vi "Main.vi"() -> ()   [LabVIEW 2013, in "LinksApplication.lvclass"]
uses:
  LinksApplication.lvclass
  System.Windows.Forms
  Featherweight/Core/Actor/Instance/FTW-Actor.lvclass
  Featherweight/Core/Actor/Reference/FTW-ActorReference.lvclass
  Featherweight/Web/Utils/FTW-Web-HTTPResponseCode.ctl
  Featherweight/Core/Actor/Instance/FTW-Actor.lvclass/FTW-Actor.ctl
  Featherweight/Core/Sequencer/FTW-Sequencer.lvclass/FTW-Sequencer.ctl
  Featherweight/Core/Sequencer/FTW-SEQ-AddNext.vi
  Featherweight/Web/Server/FTW-WebService.lvclass
  <vilib>/wsapi/Web Request.lvclass
panel:
  in  "Top Level LabVIEW File":path caption="Select a LabVIEW File (VI, LVClass, LVLib) to analyze its static linkages"
  in  "Canvas":refnum<k24>(container)
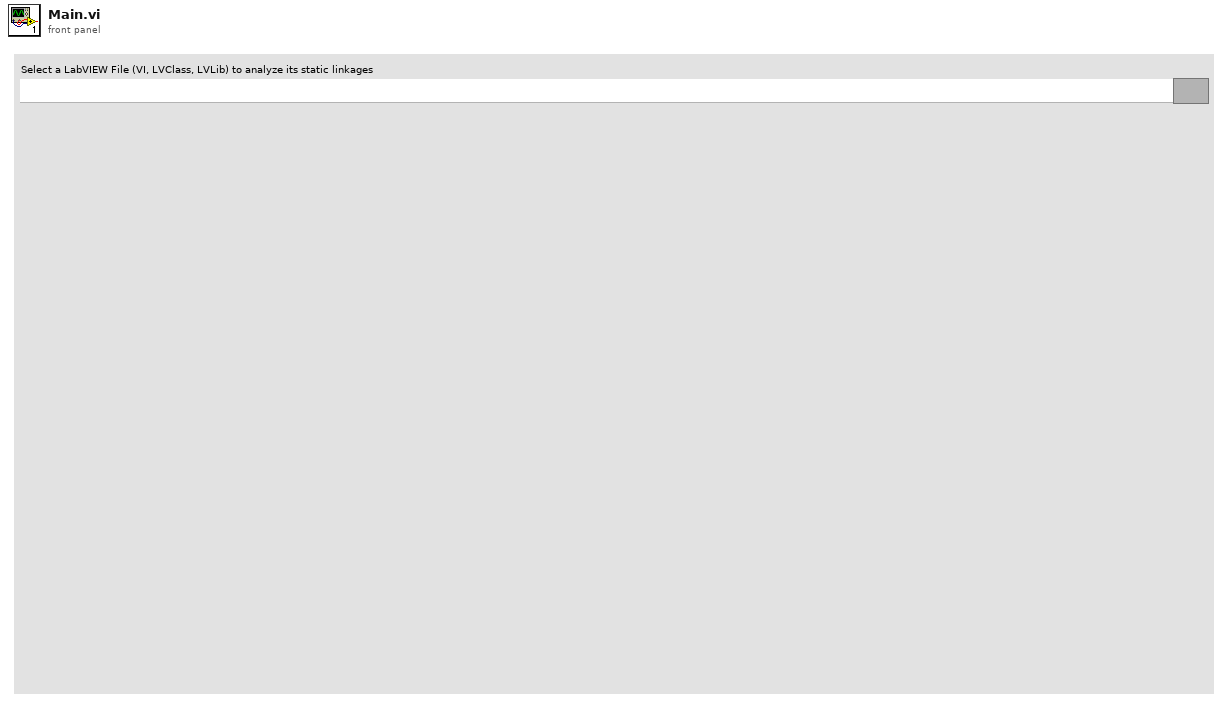
[diagram p1: front panel]
types:
  T1 = typedef "FTW-Web-HTTPResponseCode.ctl" = i32
  T2 = cluster{"Incoming HTTP Request":refnum<event-registration>}
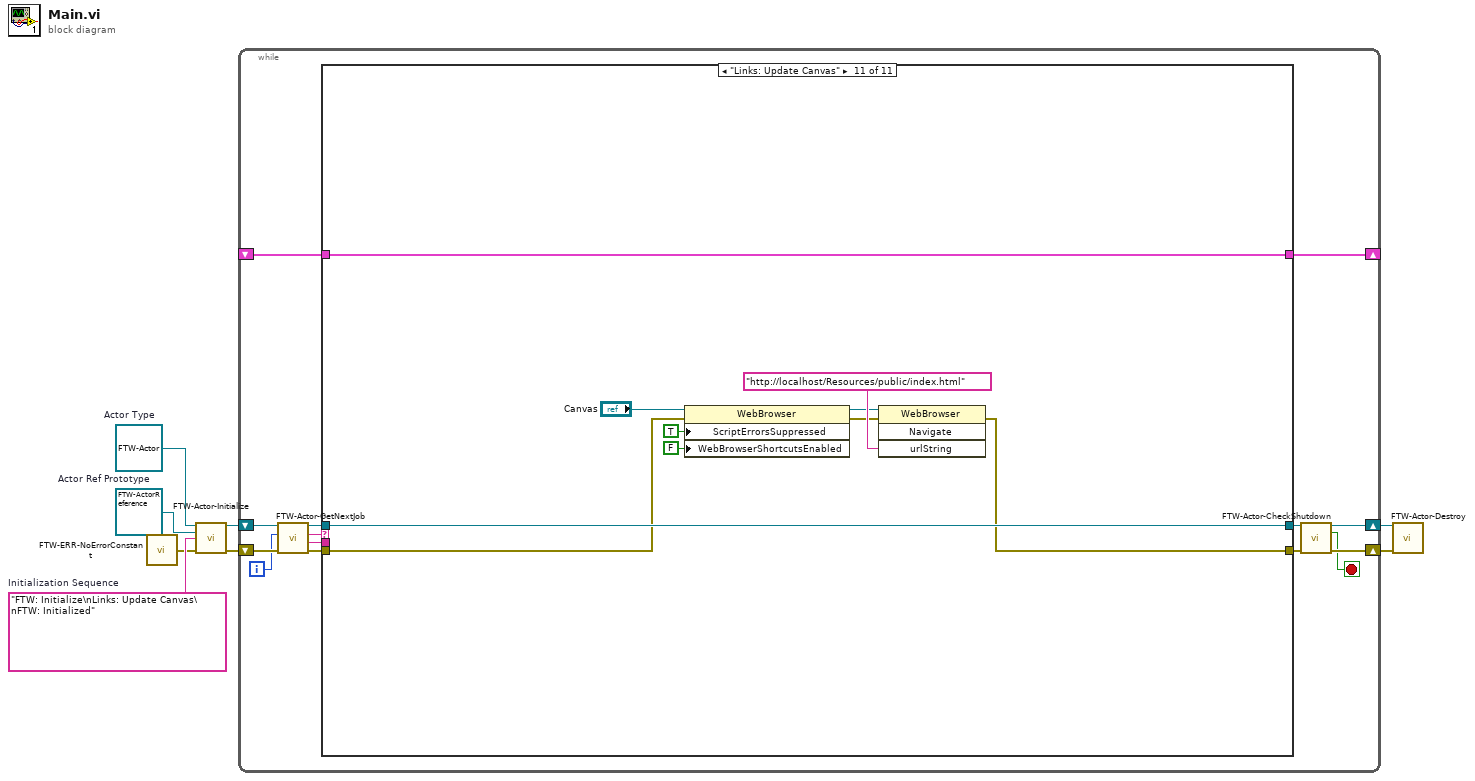
[diagram p0: block diagram]
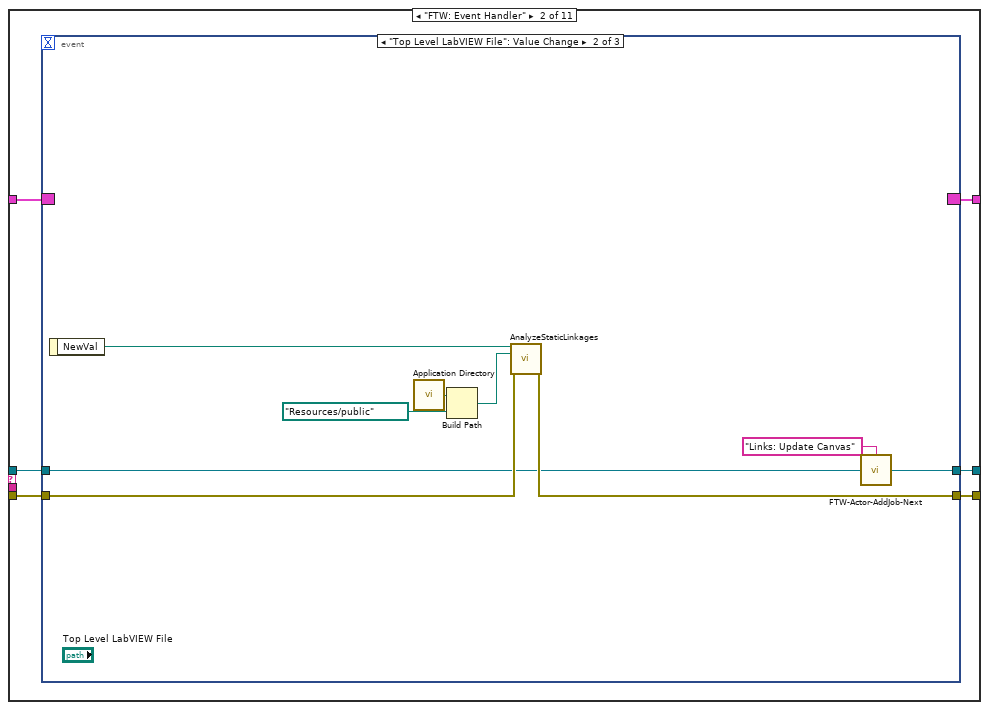
[diagram p3: hidden frame]
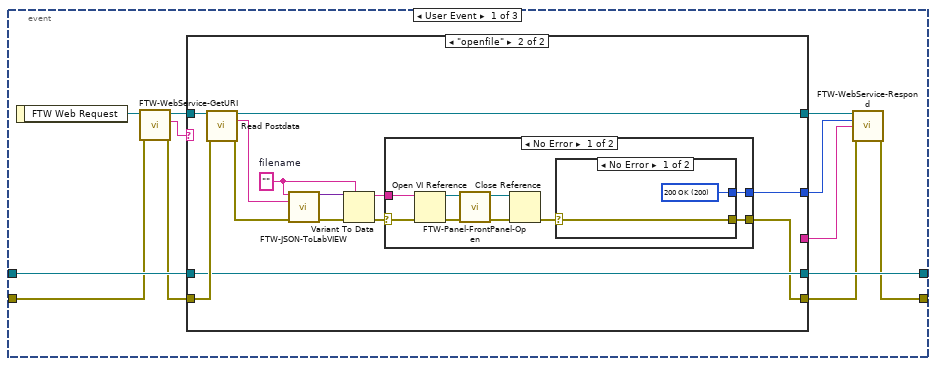
[diagram p4: hidden frame]
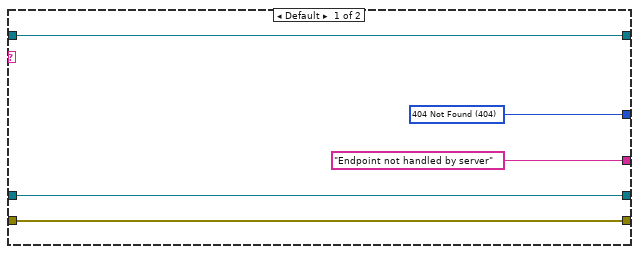
[diagram p5: hidden frame]
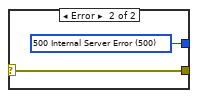
[diagram p6: hidden frame]
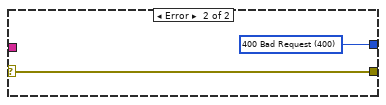
[diagram p7: hidden frame]
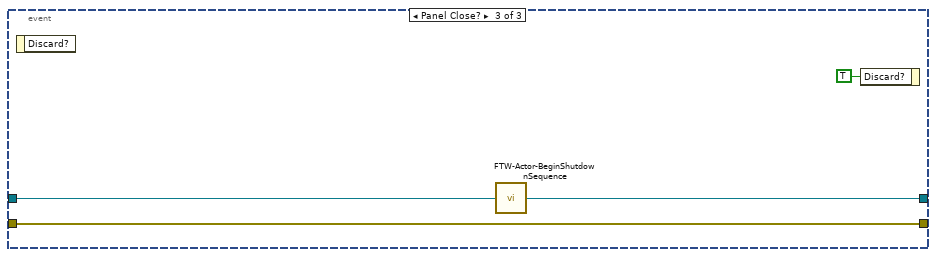
[diagram p8: hidden frame]
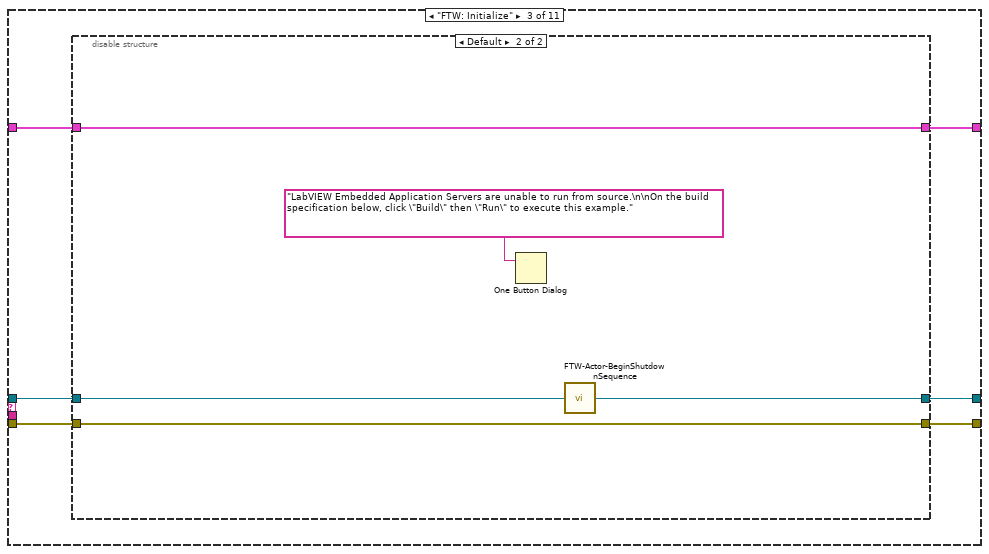
[diagram p9: hidden frame]
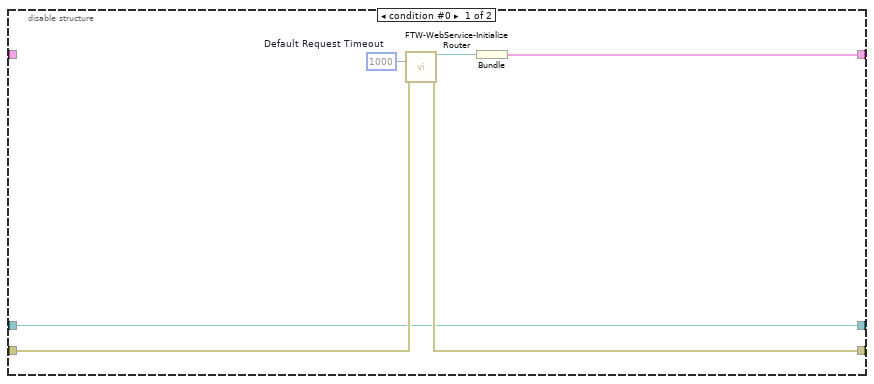
[diagram p10: hidden frame]
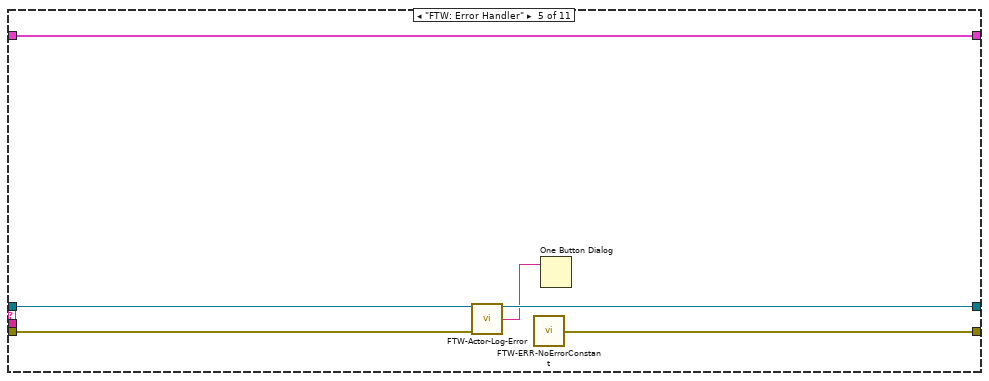
[diagram p12: hidden frame]
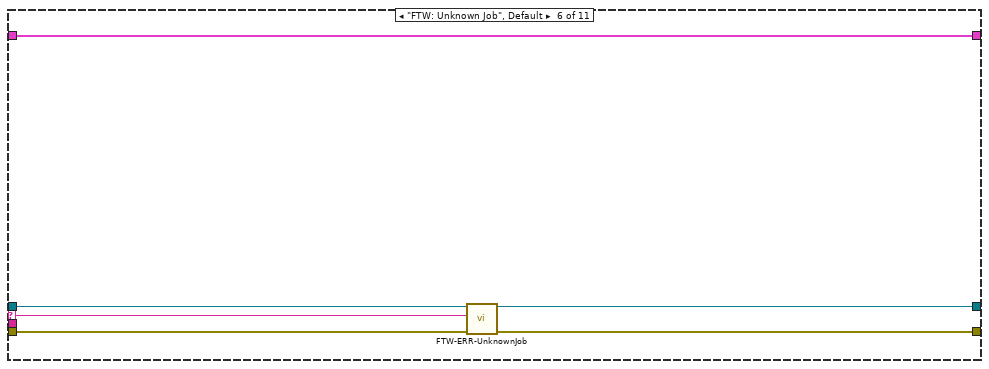
[diagram p13: hidden frame]
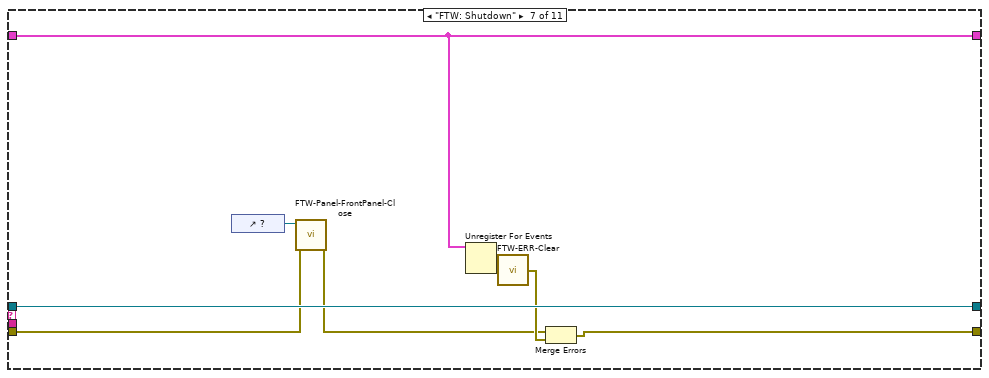
[diagram p14: hidden frame]
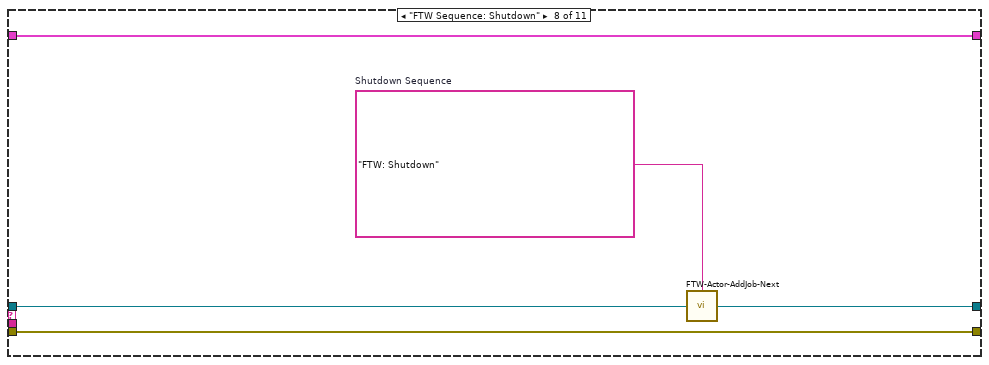
[diagram p15: hidden frame]
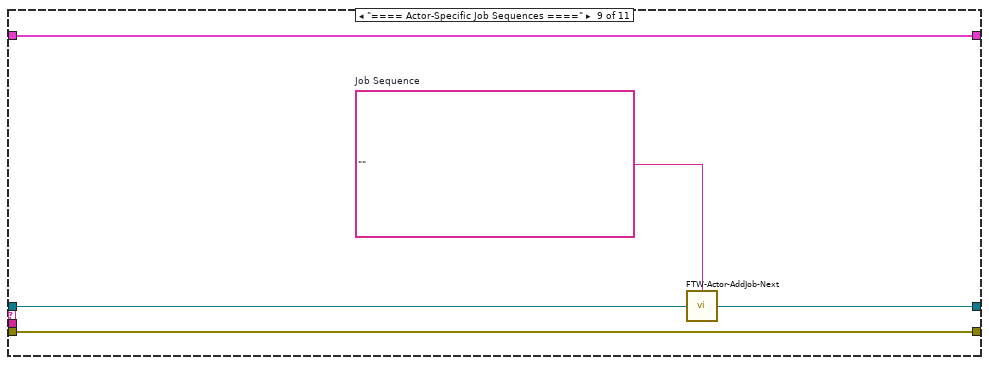
[diagram p16: hidden frame]
diagram:
  w2 = refnum<class "FTW-ActorReference.lvclass"> refnum  # Actor Ref Prototype
  w4 = refnum<class "FTW-Actor.lvclass"> refnum  # Actor Type
  w3 = "FTW: Initialize\nLinks: Update Canvas\nFTW: Initialized"  # Initialization Sequence
  n1 = call "FTW-ERR-NoErrorConstant.vi"() -> ("no error"=w1:errorcluster)
  n2 = call-dynamic "FTW-Actor-Initialize.vi"("Uninitialized FTW Actor"=w4, "Actor Ref Prototype"=w2, "Initialization Job Sequence"=w3, "error in"=w1) -> ("FTW Actor"=w8:refnum<class "FTW-Actor.lvclass">, "error out"=w5:errorcluster)  [unwired: 10 in]
  n3 = while {
    shift-right: [w12] -> w6
    shift-left: w5 -> [w19]
    shift-right: [w9] -> _
    shift-left: _ -> [w22]
    shift-right: [w14] -> w7
    shift-left: w8 -> [w21]
    i -> [w10]
    stop <- w11 stop-if-true
    n4 = call "FTW-Actor-GetNextJob.vi"("error in"=w19, "Jobs Performed"=w10, "FTW Actor in"=w21) -> ("error out"=w18:errorcluster, "Job Data"=w16:string, "Job Name"=w17:string, "FTW Actor"=w20:refnum<class "FTW-Actor.lvclass">)  [unwired: 5 in]
    n5 = case shown="\"Links: Update Canvas\"" w17 {
      selector: w17 -> [_ _ _ _ _ w116 _ _ _ _ _]
      tunnel: [w24 w31 w93 w109 w114 w117 w128 w132 w137 w141 w148] -> w13
      tunnel: w18 -> [w24 w30 w94 w109 w111 w118 w123 w132 w137 w141 w144]
      tunnel: w22 -> [w25 w28 w92 w108 w115 w120 w126 w133 w138 w140 w151]
      tunnel: [w25 w29 w95 w108 w115 w120 w126 w133 w138 w140 w151] -> w9
      tunnel: w16 -> [_ _ _ _ _ _ _ _ _ _ _]
      tunnel: [w23 w27 w91 w107 w112 w119 w127 w130 w135 w139 w150] -> w15
      tunnel: w20 -> [w23 w26 w90 w107 w113 w119 w127 w131 w136 w139 w150]
      frame "==== Featherweight Framework Jobs ====" {
      }
      frame "FTW: Event Handler" {
        n6 = event shown="[1] \"Top Level LabVIEW File\": Value Change" {
          selector: w28 -> [_ _ _]
          dyn-events: [_ _ _] -> w29
          timeout: _ -> [_ _ _]
          tunnel: [w33 w80 w88] -> w31
          tunnel: w30 -> [w40 w84 w88]
          tunnel: [w43 w78 w86] -> w27
          tunnel: w26 -> [w42 w79 w87]
          event User Event {
            n7 = event-data() -> ("FTW Web Request"=w41:refnum<class "FTW-WebService.lvclass">)  [unwired: 1 in]
            n8 = call "FTW-WebService-GetURI.vi"("error in"=w40, "FTW Web Request"=w41) -> ("error out"=w39:errorcluster, "RequestURI"=w38:string, "FTW Web Request out"=w37:refnum<class "FTW-WebService.lvclass">)  [unwired: 7 in]
            n9 = case shown="\"openfile\"" w38 {
              tunnel: [w46 w50] -> w32
              tunnel: w39 -> [w46 w60]
              tunnel: [w48 w59] -> w43
              tunnel: w42 -> [w48 w59]
              tunnel: w37 -> [w47 w61]
              tunnel: [w47 w57] -> w36
              tunnel: [w45 w58] -> w35
              tunnel: ["Endpoint not handled by server" ("Response Body") _] -> w34
              frame Default {
                w45 = T1 404 items=["100 Continue"=100, "101 Switching Protocols"=101, "200 OK"=200, "201 Created"=201, "202 Accepted"=202, "203 Non-Authoritative Information"=203, "204 No Content"=204, "205 Reset Content"=205, "206 Partial Content"=206, "300 Multiple Choices"=300, "301 Moved Permanently"=301, "302 Found"=302, "303 See Other"=303, "304 Not Modified"=304, "305 Use Proxy"=305, "306 (Unused)"=306, "307 Temporary Redirect"=307, "400 Bad Request"=400, "401 Unauthorized"=401, "402 Payment Required"=402, "403 Forbidden"=403, "404 Not Found"=404, "405 Method Not Allowed"=405, "406 Not Acceptable"=406, "407 Proxy Authentication Required"=407, "408 Request Timeout"=408, "409 Conflict"=409, "410 Gone"=410, "411 Length Required"=411, "412 Precondition Failed"=412, "413 Request Entity Too Large"=413, "414 Request-URI Too Long"=414, "415 Unsupported Media Type"=415, "416 Requested Range Not Satisfiable"=416, "417 Expectation Failed"=417, "500 Internal Server Error"=500, "501 Not Implemented"=501, "502 Bad Gateway"=502, "503 Service Unavailable"=503, "504 Gateway Timeout"=504, "505 HTTP Version Not Supported"=505] ("HTTP Response Code")
              }
              frame "openfile" {
                w53 = ""  # filename
                n10 = call <vilib>:"Read Postdata.vi"("LabVIEW Web Service Request"=w61, "error in (no error)"=w60) -> ("LabVIEW Web Service Request out"=w57:refnum<class "FTW-WebService.lvclass">, "postdata"=w56:string, "error out"=w55:errorcluster)  [unwired: 11 in]
                n11 = call "FTW-JSON-ToLabVIEW.vi"("Type and Defaults"=w53, "JSON String"=w56, "error in"=w55) -> ("Populated Values"=w54:variant, "error out"=w52:errorcluster)  [unwired: 11 in]
                n12 = Variant To Data(error in=w52, type=w53, Variant=w54) -> (data=w51:string, error out=w49:errorcluster)
                n13 = case shown="No Error" w49 {
                  selector: w49 -> [w65 w76]
                  tunnel: [w63 w75] -> w58
                  tunnel: w51 -> [w68 _]
                  tunnel: [w62 w76] -> w50
                  frame No Error {
                    n14 = Open VI Reference(vi path=w68, error in (no error)=w65) -> (vi reference=w70:refnum<vi>, error out=w69:errorcluster)  [unwired: 4 in]
                    n15 = call "FTW-Panel-FrontPanel-Open.vi"("error in"=w69, "VI Ref"=w70) -> ("error out"=w66:errorcluster, "VI Ref out"=w67:refnum<vi>)  [unwired: 8 in]
                    n16 = Close Reference(reference=w67, error in (no error)=w66) -> (error out=w64:errorcluster)
                    n17 = case shown="No Error" w64 {
                      selector: w64 -> [w71 w73]
                      tunnel: [w72 w74] -> w63
                      tunnel: [w71 w73] -> w62
                      frame No Error {
                        w72 = T1 200 items=["100 Continue"=100, "101 Switching Protocols"=101, "200 OK"=200, "201 Created"=201, "202 Accepted"=202, "203 Non-Authoritative Information"=203, "204 No Content"=204, "205 Reset Content"=205, "206 Partial Content"=206, "300 Multiple Choices"=300, "301 Moved Permanently"=301, "302 Found"=302, "303 See Other"=303, "304 Not Modified"=304, "305 Use Proxy"=305, "306 (Unused)"=306, "307 Temporary Redirect"=307, "400 Bad Request"=400, "401 Unauthorized"=401, "402 Payment Required"=402, "403 Forbidden"=403, "404 Not Found"=404, "405 Method Not Allowed"=405, "406 Not Acceptable"=406, "407 Proxy Authentication Required"=407, "408 Request Timeout"=408, "409 Conflict"=409, "410 Gone"=410, "411 Length Required"=411, "412 Precondition Failed"=412, "413 Request Entity Too Large"=413, "414 Request-URI Too Long"=414, "415 Unsupported Media Type"=415, "416 Requested Range Not Satisfiable"=416, "417 Expectation Failed"=417, "500 Internal Server Error"=500, "501 Not Implemented"=501, "502 Bad Gateway"=502, "503 Service Unavailable"=503, "504 Gateway Timeout"=504, "505 HTTP Version Not Supported"=505] ("HTTP Response Code")
                      }
                      frame Error {
                        w74 = T1 500 items=["100 Continue"=100, "101 Switching Protocols"=101, "200 OK"=200, "201 Created"=201, "202 Accepted"=202, "203 Non-Authoritative Information"=203, "204 No Content"=204, "205 Reset Content"=205, "206 Partial Content"=206, "300 Multiple Choices"=300, "301 Moved Permanently"=301, "302 Found"=302, "303 See Other"=303, "304 Not Modified"=304, "305 Use Proxy"=305, "306 (Unused)"=306, "307 Temporary Redirect"=307, "400 Bad Request"=400, "401 Unauthorized"=401, "402 Payment Required"=402, "403 Forbidden"=403, "404 Not Found"=404, "405 Method Not Allowed"=405, "406 Not Acceptable"=406, "407 Proxy Authentication Required"=407, "408 Request Timeout"=408, "409 Conflict"=409, "410 Gone"=410, "411 Length Required"=411, "412 Precondition Failed"=412, "413 Request Entity Too Large"=413, "414 Request-URI Too Long"=414, "415 Unsupported Media Type"=415, "416 Requested Range Not Satisfiable"=416, "417 Expectation Failed"=417, "500 Internal Server Error"=500, "501 Not Implemented"=501, "502 Bad Gateway"=502, "503 Service Unavailable"=503, "504 Gateway Timeout"=504, "505 HTTP Version Not Supported"=505] ("HTTP Response Code")
                      }
                    }
                  }
                  frame Error {
                    w75 = T1 400 items=["100 Continue"=100, "101 Switching Protocols"=101, "200 OK"=200, "201 Created"=201, "202 Accepted"=202, "203 Non-Authoritative Information"=203, "204 No Content"=204, "205 Reset Content"=205, "206 Partial Content"=206, "300 Multiple Choices"=300, "301 Moved Permanently"=301, "302 Found"=302, "303 See Other"=303, "304 Not Modified"=304, "305 Use Proxy"=305, "306 (Unused)"=306, "307 Temporary Redirect"=307, "400 Bad Request"=400, "401 Unauthorized"=401, "402 Payment Required"=402, "403 Forbidden"=403, "404 Not Found"=404, "405 Method Not Allowed"=405, "406 Not Acceptable"=406, "407 Proxy Authentication Required"=407, "408 Request Timeout"=408, "409 Conflict"=409, "410 Gone"=410, "411 Length Required"=411, "412 Precondition Failed"=412, "413 Request Entity Too Large"=413, "414 Request-URI Too Long"=414, "415 Unsupported Media Type"=415, "416 Requested Range Not Satisfiable"=416, "417 Expectation Failed"=417, "500 Internal Server Error"=500, "501 Not Implemented"=501, "502 Bad Gateway"=502, "503 Service Unavailable"=503, "504 Gateway Timeout"=504, "505 HTTP Version Not Supported"=505] ("HTTP Response Code")
                  }
                }
              }
            }
            n18 = call "FTW-WebService-Respond.vi"("FTW Web Request"=w36, "HTTP Response Code"=w35, "Response Body"=w34, "error in"=w32) -> ("error out"=w33:errorcluster)  [unwired: 10 in, 1 out]
          }
          event "Top Level LabVIEW File": Value Change {
            n19 = event-data() -> ("NewVal"=w85:path)  [unwired: 1 in]
            n20 = call <vilib>:"Application Directory.vi"() -> ("Application Directory"=w83:path)
            n21 = Build Path(base path=w83, name or relative path=path "Resources/public") -> (appended path=w82:path)
            n22 = call "AnalyzeStaticLinkages.vi"("LabVIEW File to Analyze"=w85, "Public Server Directory"=w82, "error in"=w84) -> ("error out"=w80:errorcluster)  [unwired: 12 in]
            n23 = call "FTW-Actor-AddJob-Next.vi"("Add Next in Job Queue"="Links: Update Canvas", "FTW Actor"=w79) -> ("FTW Actor out"=w78:refnum<class "FTW-Actor.lvclass">)  [unwired: 2 in]
          }
          event Panel Close? {
            n24 = event-data() -> ()  [unwired: 1 in, 1 out]
            n25 = call "FTW-Actor-BeginShutdownSequence.vi"("FTW Actor"=w87) -> ("FTW Actor out"=w86:refnum<class "FTW-Actor.lvclass">)  [unwired: 3 in]
            n26 = event-data("Discard?"=TRUE) -> ()  [unwired: 1 in, 1 out]
          }
        }
      }
      frame "FTW: Initialize" {
        n27 = disable-structure shown="Default" {
          disable-tunnel: [w101 w106] -> w95
          disable-tunnel: w94 -> [w98 w103]
          disable-tunnel: [w97 w103] -> w93
          disable-tunnel: w92 -> [_ w106]
          disable-tunnel: [w96 w104] -> w91
          disable-tunnel: w90 -> [w96 w105]
          frame condition #0 {
            w99 = 1000  # Default Request Timeout
            n28 = call "FTW-WebService-InitializeRouter.vi"("Default Request Timeout"=w99, "error in"=w98) -> ("Incoming HTTP Request"=w100:refnum<event-registration>, "error out"=w97:errorcluster)  [unwired: 12 in]
            n29 = Bundle("Incoming HTTP Request"=w100) -> (w101:T2)  [unwired: 1 in]
          }
          frame condition #1 (active) {
            n30 = One Button Dialog(message="LabVIEW Embedded Application Servers are unable to run from source.\n\nOn the build specification below, click \"Build\" then \"Run\" to execute this example.") -> ()  [unwired: 1 in, 1 out]
            n31 = call "FTW-Actor-BeginShutdownSequence.vi"("FTW Actor"=w105) -> ("FTW Actor out"=w104:refnum<class "FTW-Actor.lvclass">)  [unwired: 3 in]
          }
        }
      }
      frame "FTW: Initialized" {
      }
      frame "FTW: Error Handler" {
        n32 = call-dynamic "FTW-Actor-Log-Error.vi"("Featherweight Actor"=w113, "Error to Log"=w111) -> ("Featherweight Actor out"=w112:refnum<class "FTW-Actor.lvclass">, "Serialized Event"=w110:string)  [unwired: 11 in, 1 out]
        n33 = call "FTW-ERR-NoErrorConstant.vi"() -> ("no error"=w114:errorcluster)
        n34 = One Button Dialog(message=w110) -> ()  [unwired: 1 in, 1 out]
      }
      frame "FTW: Unknown Job", Default {
        n35 = call "FTW-ERR-UnknownJob.vi"("error in"=w118, "Unknown Job"=w116) -> ("error out"=w117:errorcluster)  [unwired: 9 in]
      }
      frame "FTW: Shutdown" {
        n36 = control-ref of="?"() -> (w121:refnum<vi>)
        n37 = call "FTW-Panel-FrontPanel-Close.vi"("error in"=w123, "VI Ref"=w121) -> ("error out"=w122:errorcluster)  [unwired: 8 in, 1 out]
        n38 = Unregister For Events(event registration refnum=w126) -> (error out=w125:errorcluster)  [unwired: 1 in]
        n39 = call "FTW-ERR-Clear.vi"("error to snuff"=w125) -> ("no error"=w124:errorcluster)
        n40 = Merge Errors(w122, w124) -> (w128:errorcluster)
      }
      frame "FTW Sequence: Shutdown" {
        w129 = "FTW: Shutdown"  # Shutdown Sequence
        n41 = call "FTW-Actor-AddJob-Next.vi"("Add Next in Job Queue"=w129, "FTW Actor"=w131) -> ("FTW Actor out"=w130:refnum<class "FTW-Actor.lvclass">)  [unwired: 2 in]
      }
      frame "==== Actor-Specific Job Sequences ====" {
        w134 = ""  # Job Sequence
        n42 = call "FTW-Actor-AddJob-Next.vi"("Add Next in Job Queue"=w134, "FTW Actor"=w136) -> ("FTW Actor out"=w135:refnum<class "FTW-Actor.lvclass">)  [unwired: 2 in]
      }
      frame "==== Actor-Specific Jobs ====" {
      }
      frame "Links: Update Canvas" {
        n43 = property class="WebBrowser"(reference="Canvas", error in=w144, "ScriptErrorsSuppressed"=TRUE, "WebBrowserShortcutsEnabled"=FALSE) -> (reference out=w142:refnum<k24>, error out=w143:errorcluster)
        n44 = invoke class="WebBrowser" method="Navigate"(reference=w142, error in=w143, "urlString"="http://localhost/Resources/public/index.html") -> (error out=w148:errorcluster)  [unwired: 1 in, 3 out]
      }
    }
    n45 = call "FTW-Actor-CheckShutdown.vi"("FTW Actor in"=w15, "error in"=w13) -> ("FTW Actor"=w14:refnum<class "FTW-Actor.lvclass">, "Shutdown?"=w11:bool, "error out"=w12:errorcluster)  [unwired: 11 in]
  }
  n46 = call-dynamic "FTW-Actor-Destroy.vi"("FTW Actor"=w7, "error in"=w6) -> ()  [unwired: 13 in, 1 out]
